vi "close.vi"(8 "error in (no error)":errorcluster caption="错误输入（无错误）", 11 "serial 输入":refnum<class "serial.lvclass">) -> (0 "error out":errorcluster caption="错误输出", 3 "serial 输出":refnum<class "serial.lvclass">)   [LabVIEW 2016, in "潮位站数据传输.lvlib" / "serial.lvclass"]
uses:
  serial.lvclass
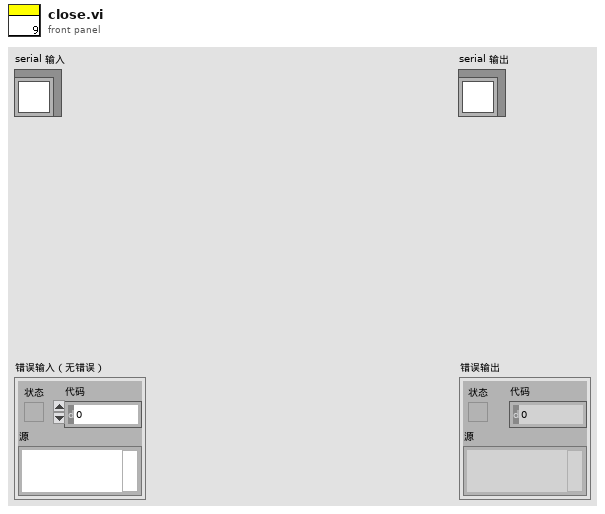
[diagram p1: front panel]
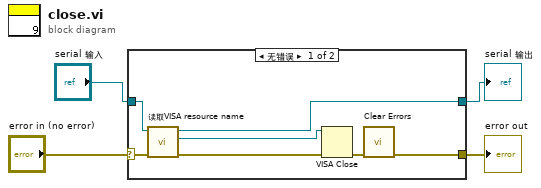
[diagram p0: block diagram]
diagram:
  n1 = case shown="无错误" "error in (no error)" {
    selector: "error in (no error)" -> [w10 w12]
    tunnel: "serial 输入" -> [w11 w13]
    tunnel: [w8 w12] -> w2
    tunnel: [w5 w13] -> w1
    frame No Error {
      n2 = call-dynamic "读取VISA resource name.vi"("error in (no error)"=w10, "data_inter输入"=w11) -> ("error out"=w7:errorcluster, "VISA resource name"=w6:refnum<visa-resource-name>, "data_inter输出"=w5:refnum<class "serial.lvclass">)  [unwired: 7 in]
      n3 = VISA Close(VISA resource name=w6, error in (no error)=w7) -> (error out=w9:errorcluster)
      n4 = call <vilib>:"Clear Errors.vi"("error in (no error)"=w9) -> ("error out"=w8:errorcluster)  [unwired: 5 in, 1 out]
    }
    frame Error {
    }
  }
  "error out" <- w2
  "serial 输出" <- w1
